vi "Open LED.vi"(8 "DIO Channel Red":T1, 9 "DIO Channel Green":T1, 10 "DIO Channel Blue":T1, 11 "refnum name":string) -> (3 "Light refnum":string)   [LabVIEW 2016]
uses:
  <vilib>/Rock Robotics/SystemInterfaces/DIO/FPGA_DIOChannel.ctl
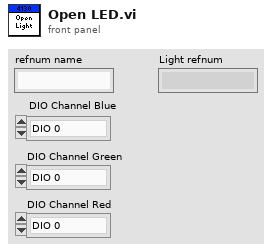
[diagram p1: front panel]
types:
  T1 = typedef "FPGA_DIOChannel.ctl" = enum8{"DIO 0", "DIO 1", "DIO 2", "DIO 3", "DIO 4", "DIO 5", "DIO 6", "DIO 7", "DIO 8", "DIO 9", "DIO MXP 0", "DIO MXP 1", "DIO MXP 2", "DIO MXP 3", "DIO MXP 4", "DIO MXP 5", "DIO MXP 6", "DIO MXP 7", "DIO MXP 8", "DIO MXP 9", "DIO MXP 10", "DIO MXP 11", "DIO MXP 12", "DIO MXP 13", "DIO MXP 14", "DIO MXP 15", "SPI Port CS1", "SPI Port CS2", "SPI Port CS3", "SPI Port MISO", "SPI Port MOSI", "Invalid"}
  T2 = typedef "WPI_DigitalOutputDevRef.ctl" = cluster{"DIO Channel":T1, "DevStatus":errorcluster}
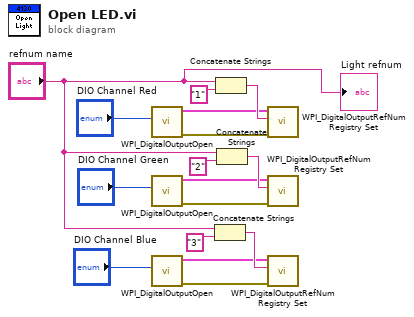
[diagram p0: block diagram]
diagram:
  n1 = call <vilib>:"WPI_DigitalOutputOpen.vi"("DIO Channel"="DIO Channel Red") -> ("error out"=w2:errorcluster, "DigitalOutputDevRef"=w3:T2)  [unwired: 9 in]
  n2 = call <vilib>:"WPI_DigitalOutputOpen.vi"("DIO Channel"="DIO Channel Green") -> ("error out"=w10:errorcluster, "DigitalOutputDevRef"=w9:T2)  [unwired: 9 in]
  n3 = call <vilib>:"WPI_DigitalOutputOpen.vi"("DIO Channel"="DIO Channel Blue") -> ("error out"=w11:errorcluster, "DigitalOutputDevRef"=w12:T2)  [unwired: 9 in]
  n4 = Concatenate Strings("refnum name", "3" ("string")) -> (w14:string)
  n5 = Concatenate Strings("refnum name", "1" ("string")) -> (w16:string)
  n6 = Concatenate Strings("refnum name", "2" ("string")) -> (w15:string)
  n7 = call <vilib>:"WPI_DigitalOutputRefNum Registry Set.vi"("error in (no error)"=w2, "refnum name"=w16, "DigitalOutputDevRef"=w3) -> ()  [unwired: 7 in, 2 out]
  n8 = call <vilib>:"WPI_DigitalOutputRefNum Registry Set.vi"("error in (no error)"=w10, "refnum name"=w15, "DigitalOutputDevRef"=w9) -> ()  [unwired: 7 in, 2 out]
  n9 = call <vilib>:"WPI_DigitalOutputRefNum Registry Set.vi"("error in (no error)"=w11, "refnum name"=w14, "DigitalOutputDevRef"=w12) -> ()  [unwired: 7 in, 2 out]
  "Light refnum" <- "refnum name"
